vi "DecodeMonitorHeader(EntrySize).vi"(11 "EntrySizeWord":u32 format="%.0x") -> (3 "EntrySize":T1)   [LabVIEW 2020, in "AIM664LV.lvlib"]
uses:
  AIM664LV.lvlib
  _controls/monitor_entrySize_type.ctl
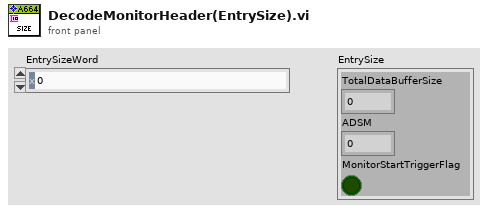
[diagram p1: front panel]
types:
  T1 = typedef "AIM664LV.lvlib/monitor_entrySize_type.ctl" = cluster{"TotalDataBufferSize":u16, "ADSM":u16, "MonitorStartTriggerFlag":bool}
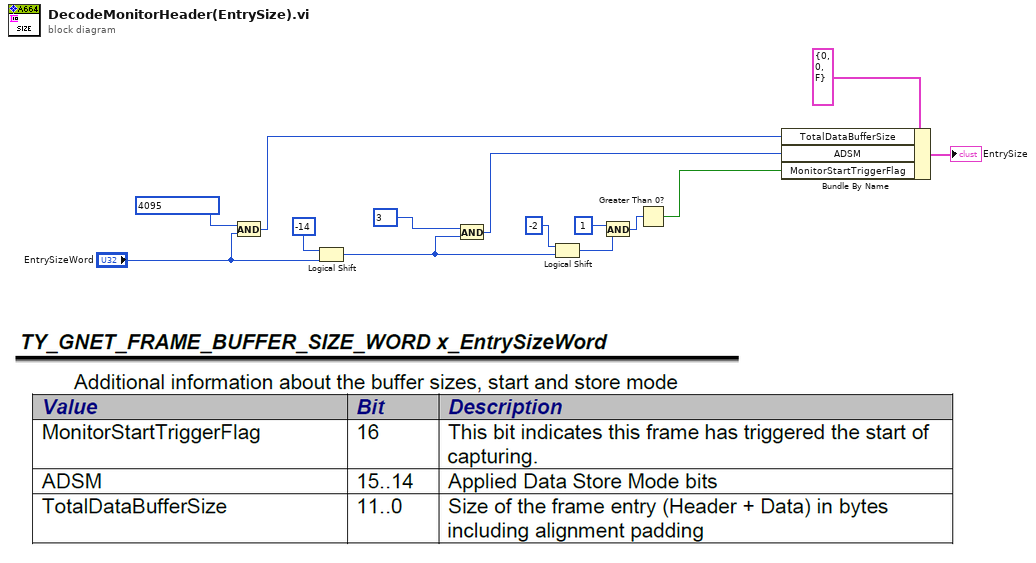
[diagram p0: block diagram]
diagram:
  n1 = And(x=u32 4095 ("Numeric"), y="EntrySizeWord") -> (x .and. y?=w3:u32)
  n2 = Logical Shift(y=i16 -14, x="EntrySizeWord") -> (x << y=w8:u32)
  n3 = And(x=u32 3 ("Numeric"), y=w8) -> (x .and. y?=w2:u32)
  n4 = Logical Shift(y=i16 -2, x=w8) -> (x << y=w6:u32)
  n5 = And(x=u32 1 ("Numeric"), y=w6) -> (x .and. y?=w7:u32)
  n6 = Greater Than 0?(x=w7) -> (x > 0?=w1:bool)
  n7 = Bundle By Name(cluster=T1 {"TotalDataBufferSize"=0, "ADSM"=0, "MonitorStartTriggerFlag"=FALSE} ("FHW1"), "TotalDataBufferSize"=w3, "ADSM"=w2, "MonitorStartTriggerFlag"=w1) -> (→"EntrySize":T1)
